vi "close MB.vi"(8 "error in (no error)":errorcluster caption="错误输入（无错误）", 11 "MB_Serial session":refnum<class "MB_Master_Serial.lvclass">) -> (0 "error out":errorcluster caption="错误输出")   [LabVIEW 2016, in "斯坦道多参数.lvlib"]
uses:
  <vilib>/Plasmionique/MB Master/MB_Master_Serial/MB_Master_Serial.lvclass
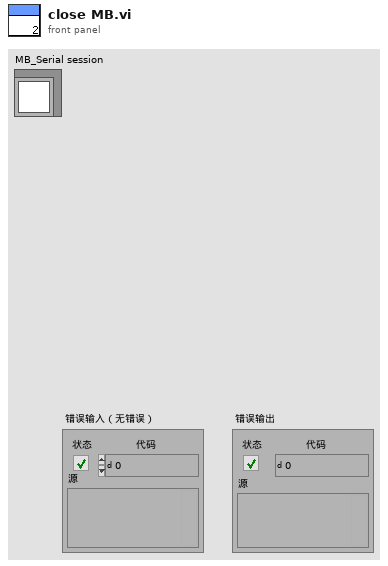
[diagram p1: front panel]
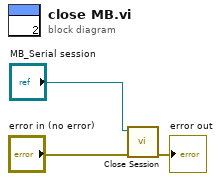
[diagram p0: block diagram]
diagram:
  n1 = call-dynamic "Close Session.vi"("error in (no error)"="error in (no error)", "MB_Serial session"="MB_Serial session") -> ("error out"=→"error out":errorcluster)  [unwired: 9 in]
